vi "I2C LCD.vi"() -> ()   [LabVIEW 2023, in "CTI-Visa-Scratchpad.lvlib"]
uses:
  CTI-Visa-Scratchpad.lvlib
  CTI-Visa-DeviceLib/LCD-I2C/LCD Size.ctl
  CTI-Visa/I2C Options.ctl
  CTI-Visa/CTI-Visa.lvlib
  CTI-Visa-DeviceLib/LCD-I2C/LCD-I2C.lvclass
panel:
  out "error out":errorcluster
  in  "Port":refnum<visa-resource-name>="COM4"
  in  "String":string="Hello LabVIEW!"
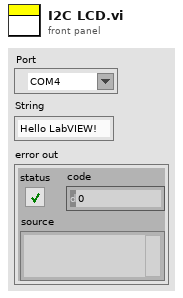
[diagram p1: front panel]
types:
  T1 = typedef "CTI-Visa.lvlib/I2C Options.ctl" = cluster{"Bus":u8, "Baud":u32, "SCL GPIO":i32, "SDA GPIO":i32}
  T2 = typedef "CTI-Visa-DeviceLib.lvlib/LCD-I2C.lvclass/LCD Size.ctl" = cluster{"Rows":u8, "Cols":u8}
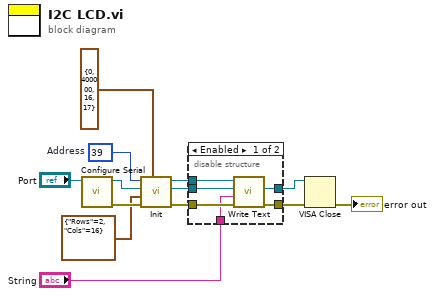
[diagram p0: block diagram]
diagram:
  w9 = u8 39  # Address
  n1 = call "Configure Serial.vi"("VISA resource name in"="Port") -> ("error out"=w11:errorcluster, "VISA resource name"=w12:refnum<visa-resource-name>)  [unwired: 9 in]
  n2 = call "Init.vi"("I2C Options"=T1 {"Bus"=0, "Baud"=400000, "SCL GPIO"=16, "SDA GPIO"=17}, "error in (no error)"=w11, "LCD Size"=T2 {"Rows"=2, "Cols"=16}, "VISA resource name in"=w12, "Address"=w9) -> ("error out"=w6:errorcluster, "VISA resource name"=w5:refnum<visa-resource-name>, "LCD-I2C out"=w7:refnum<class "LCD-I2C.lvclass">)  [unwired: 4 in]
  n3 = disable-structure shown="Enabled" {
    disable-tunnel: w7 -> [w19 _]
    disable-tunnel: w6 -> [w18 w20]
    disable-tunnel: w5 -> [w17 w21]
    disable-tunnel: "String" -> [w16 _]
    disable-tunnel: [w15 w20] -> w3
    disable-tunnel: [w14 w21] -> w2
    frame Enabled {
      n4 = call "Write Text.vi"("error in (no error)"=w18, "Text"=w16, "VISA resource name in"=w17, "LCD-I2C in"=w19) -> ("error out"=w15:errorcluster, "VISA resource name"=w14:refnum<visa-resource-name>)  [unwired: 5 in, 1 out]
    }
    frame Disabled {
    }
  }
  n5 = VISA Close(VISA resource name=w2, error in (no error)=w3) -> (error out=→"error out":errorcluster)
